vi "Call API By Path.vi"(4 "Read Data? (F)":bool, 5 "Host Resources":T1, 6 "Write Data? (F)":bool, 7 "vi path":path, 8 "error in":errorcluster, 9 "Diagnostics Queue":refnum<queue>, 10 "Generated Data":string, 11 "Hardware Configuration in":T5) -> (0 "error out":errorcluster, 2 "Acquired Data":T4, 3 "Hardware Configuration out":T5)   [LabVIEW 2021, in "Acquisition.lvlib"]
doc: "Run a VI dynamically by calling it by path.\n\nThis VI opens a reference to the target VI specified in 'vi path' and sets the target VI's inputs for 'Hardware Configuration in' and 'error in'. If 'Write Data?' is TRUE, then the 'Generated Data' input is also set on the target VI.\n\nAfter the target VI finishes executing, this VI gets the target VI's outputs for 'Hardware Configuration out' and 'error out'. If 'Read Data?' is TRUE, then the 'Acquired Data' output is also returned from the target VI."
uses:
  Acquisition.lvlib
  Hardware Configuration.ctl
  Channel Settings.ctl
  IO Device.ctl
  Sensor Type.ctl
  Interval Timer/Repeat Interval.ctl
  Interval Timer/Interval Length.ctl
  Interval Timer/Interval Token.ctl
  IO Context.ctl
  IO API.ctl
  Acquired Data.ctl
  Host Resources.ctl
  Host Software Package.ctl
  Host IO Resource.ctl
  support/Message Queue/Message Cluster.ctl
  Interval Timer/Interval Timer.lvlib
  support/Message Queue/Message Queue.lvlib
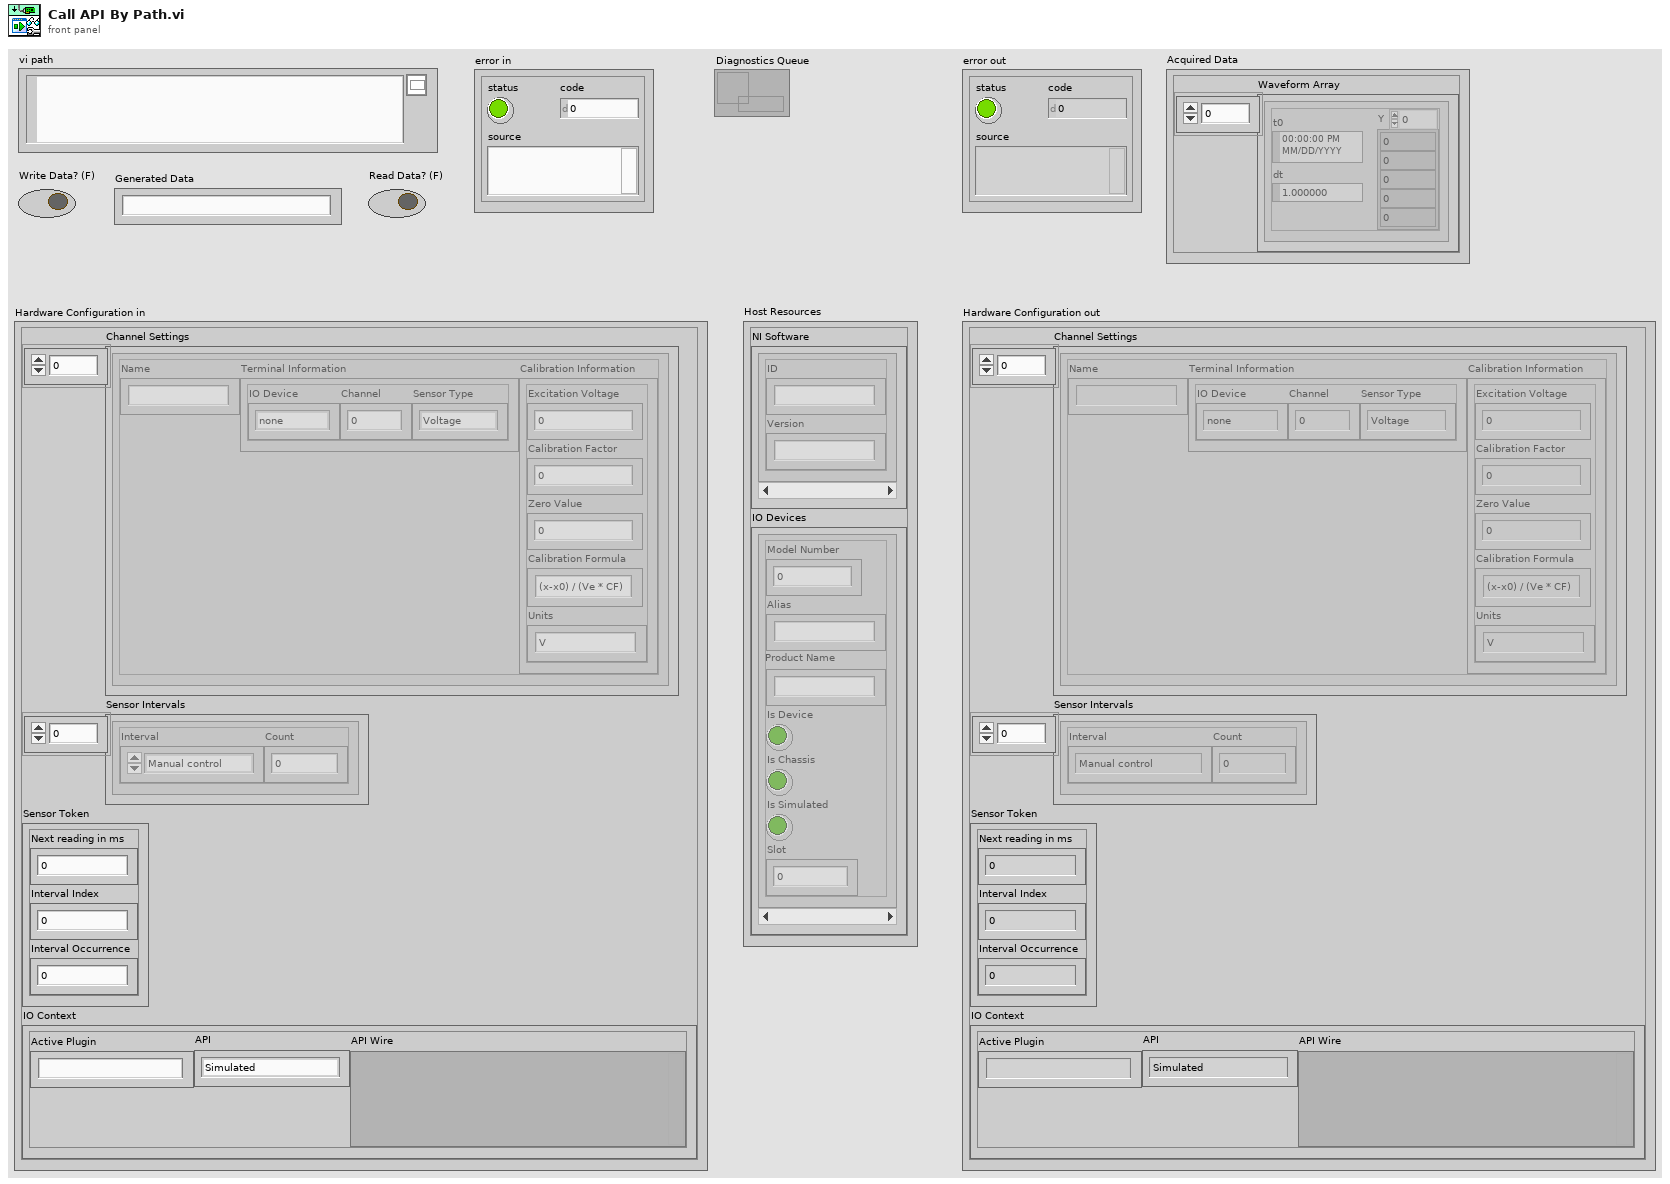
[diagram p1: front panel]
types:
  T1 = typedef "Acquisition.lvlib/Host Resources.ctl" = cluster{"NI Software":T2[], "IO Devices":T3[]}
  T2 = typedef "Acquisition.lvlib/Host Software Package.ctl" = cluster{"ID":string, "Version":string}
  T3 = typedef "Acquisition.lvlib/Host IO Resource.ctl" = cluster{"Model Number":u32, "Alias":string, "Product Name":string, "Is Device":bool, "Is Chassis":bool, "Is Simulated":bool, "Slot":i32}
  T4 = typedef "Acquisition.lvlib/Acquired Data.ctl" = cluster{"Waveform Array":waveform(dbl)[]}
  T5 = typedef "Acquisition.lvlib/Hardware Configuration.ctl" = cluster{"Channel Settings":T6[], "Sensor Intervals":T9[], "Sensor Token":T11, "IO Context":T12}
  T6 = typedef "Acquisition.lvlib/Channel Settings.ctl" = cluster{"Name":string, "Terminal Information":cluster{"IO Device":T7, "Channel":i32, "Sensor Type":T8}, "Calibration Information":cluster{"Excitation Voltage":dbl, "Calibration Factor":dbl, "Zero Value":dbl, "Calibration Formula":string, "Units":string}}
  T7 = typedef "Acquisition.lvlib/IO Device.ctl" = enum16{"none", "9219", "9401"}
  T8 = typedef "Acquisition.lvlib/Sensor Type.ctl" = enum16{"Voltage", "Load", "Pressure", "Encoder"}
  T9 = typedef "Interval Timer.lvlib/Repeat Interval.ctl" = cluster{"Interval":T10, "Count":i32}
  T10 = typedef "Interval Timer.lvlib/Interval Length.ctl" = enum16{"Manual control", "1 second", "10 seconds", "30 seconds", "60 seconds", "600 seconds", "1200 seconds", "3600 seconds"}
  T11 = typedef "Interval Timer.lvlib/Interval Token.ctl" = cluster{"Next reading in ms":u32, "Interval Index":i32, "Interval Occurrence":i32}
  T12 = typedef "Acquisition.lvlib/IO Context.ctl" = cluster{"Active Plugin":string, "API":T13, "API Wire":variant}
  T13 = typedef "Acquisition.lvlib/IO API.ctl" = enum16{"Simulated", "DAQmx"}
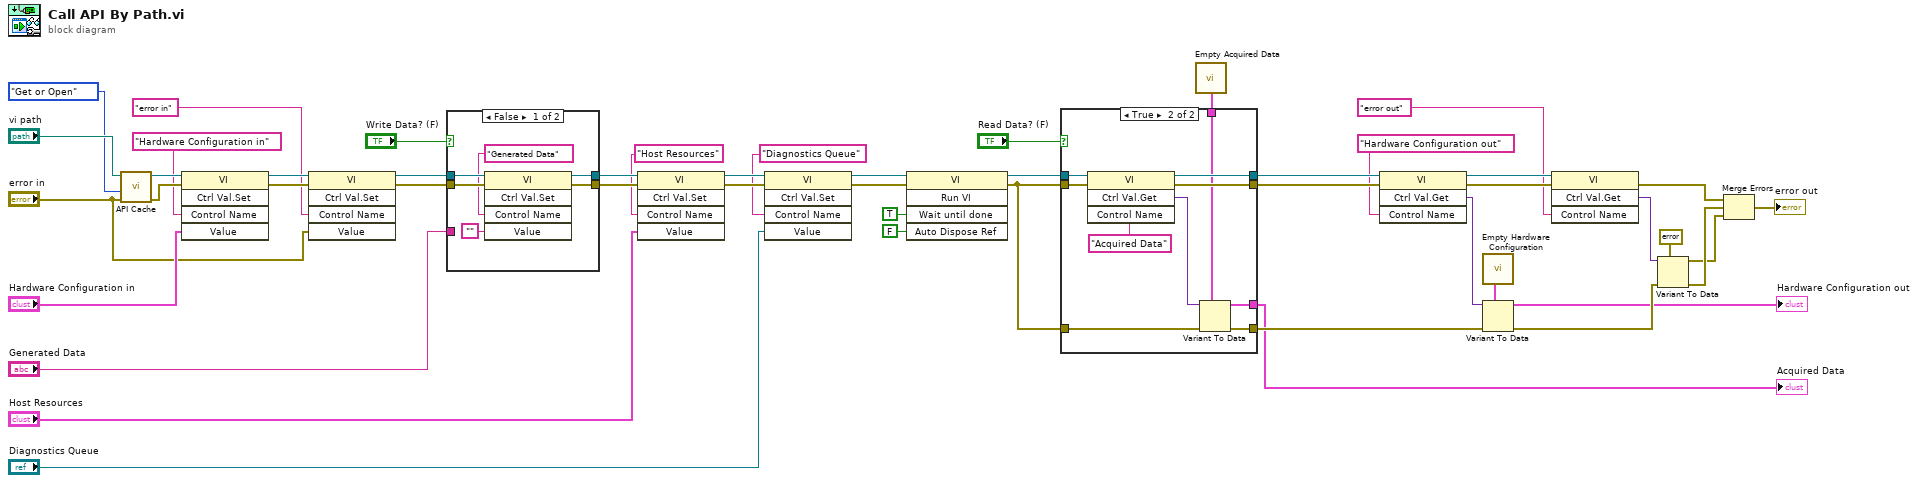
[diagram p0: block diagram]
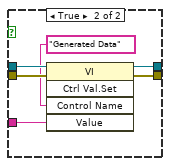
[diagram p2: hidden frame]
diagram:
  n1 = call "API Cache.vi"("error in"="error in", "Action"=enum16{"Initialize", "Get or Open", "Clear"}."Get or Open", "VI Path"="vi path") -> ("error out"=w5:errorcluster, "VI Reference"=w4:refnum<vi>)  [unwired: 7 in]
  n2 = invoke class="VI" method="Ctrl Val.Set"(reference=w4, error in=w5, "Control Name"="Hardware Configuration in", "Value"="Hardware Configuration in") -> (reference out=w48:refnum<vi>, error out=w46:errorcluster)  [unwired: 1 in, 3 out]
  n3 = invoke class="VI" method="Ctrl Val.Set"(reference=w48, error in=w46, "Control Name"="error in", "Value"="error in") -> (reference out=w22:refnum<vi>, error out=w21:errorcluster)  [unwired: 1 in, 3 out]
  n4 = case shown="False" "Write Data? (F)" {
    tunnel: w22 -> [w53 w60]
    tunnel: [w54 w59] -> w17
    tunnel: w21 -> [w52 w58]
    tunnel: [w51 w57] -> w18
    tunnel: "Generated Data" -> [_ w55]
    frame False {
      n5 = invoke class="VI" method="Ctrl Val.Set"(reference=w53, error in=w52, "Control Name"="Generated Data", "Value"="") -> (reference out=w54:refnum<vi>, error out=w51:errorcluster)  [unwired: 1 in, 3 out]
    }
    frame True {
      n6 = invoke class="VI" method="Ctrl Val.Set"(reference=w60, error in=w58, "Control Name"="Generated Data", "Value"=w55) -> (reference out=w59:refnum<vi>, error out=w57:errorcluster)  [unwired: 1 in, 3 out]
    }
  }
  n7 = invoke class="VI" method="Ctrl Val.Set"(reference=w17, error in=w18, "Control Name"="Host Resources", "Value"="Host Resources") -> (reference out=w16:refnum<vi>, error out=w15:errorcluster)  [unwired: 1 in, 3 out]
  n8 = invoke class="VI" method="Ctrl Val.Set"(reference=w16, error in=w15, "Control Name"="Diagnostics Queue", "Value"="Diagnostics Queue") -> (reference out=w13:refnum<vi>, error out=w14:errorcluster)  [unwired: 1 in, 3 out]
  n9 = invoke class="VI" method="Run VI"(reference=w13, error in=w14, "Wait until done"=TRUE ("Wait Until Done"), "Auto Dispose Ref"=FALSE ("Auto Dispose Reference")) -> (reference out=w31:refnum<vi>, error out=w26:errorcluster)  [unwired: 1 in, 3 out]
  n10 = call "Empty Acquired Data.vi"() -> ("Empty Acquired Data"=w23:T4)
  n11 = case shown="True" "Read Data? (F)" {
    tunnel: w31 -> [w64 w74]
    tunnel: [w64 w73] -> w30
    tunnel: [w63 w72] -> w29
    tunnel: w26 -> [w63 w71]
    tunnel: w26 -> [w61 w69]
    tunnel: [w61 w68] -> w25
    tunnel: [w62 w66] -> w24
    tunnel: w23 -> [w62 w65]
    frame False {
    }
    frame True {
      n12 = invoke class="VI" method="Ctrl Val.Get"(reference=w74, error in=w71, "Control Name"="Acquired Data") -> (reference out=w73:refnum<vi>, error out=w72:errorcluster, "Get Control Value Variant"=w67:variant)  [unwired: 1 in, 1 out]
      n13 = Variant To Data(error in=w69, type=w65, Variant=w67) -> (data=w66:T4, error out=w68:errorcluster)
    }
  }
  "Acquired Data" <- w24
  n14 = invoke class="VI" method="Ctrl Val.Get"(reference=w30, error in=w29, "Control Name"="Hardware Configuration out") -> (reference out=w47:refnum<vi>, error out=w45:errorcluster, "Get Control Value Variant"=w38:variant)  [unwired: 1 in, 1 out]
  n15 = call "Empty Hardware Configuration.vi"() -> ("Hardware Configuration"=w39:T5)
  n16 = Variant To Data(error in=w25, type=w39, Variant=w38) -> (data=→"Hardware Configuration out":T5, error out=w37:errorcluster)
  n17 = invoke class="VI" method="Ctrl Val.Get"(reference=w47, error in=w45, "Control Name"="error out") -> (error out=w1:errorcluster, "Get Control Value Variant"=w41:variant)  [unwired: 1 in, 2 out]
  n18 = Variant To Data(error in=w37, type=errorcluster {"status"=FALSE, "code"=0, "source"=""} ("error constant"), Variant=w41) -> (data=w33:errorcluster, error out=w36:errorcluster)
  n19 = Merge Errors(w1, w36, w33) -> (→"error out":errorcluster)
